vi "Start New File.vi"(8 "error in (no error)":errorcluster, 11 "Logger in":refnum<class "Logger.lvclass">) -> (0 "error out":errorcluster, 2 "File Path":path, 3 "Logger out":refnum<class "Logger.lvclass">)   [LabVIEW 2016, in "Logger.lvclass"]
uses:
  Logger.lvclass
  Logger.lvclass/Logger.ctl
  Read File.lvclass.vi
  Write File.lvclass.vi
  NHMFL_Core/Libraries/File/File Class/File.lvclass
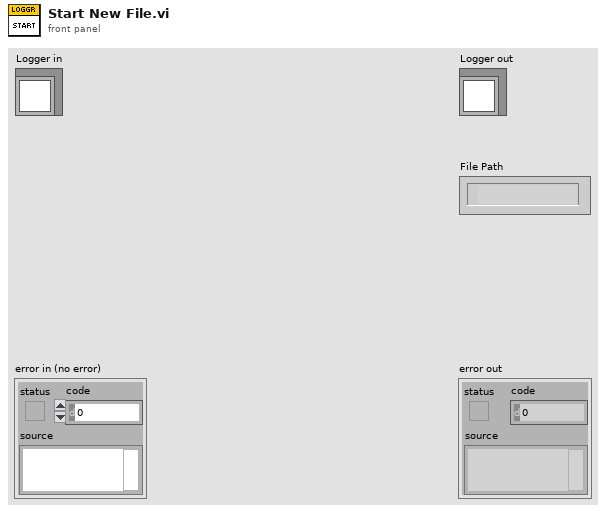
[diagram p1: front panel]
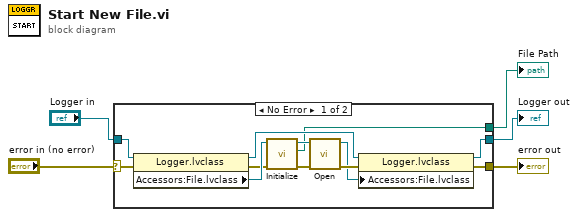
[diagram p0: block diagram]
diagram:
  n1 = case shown="No Error" "error in (no error)" {
    selector: "error in (no error)" -> [w17 w19]
    tunnel: [w12 w19] -> w4
    tunnel: [w11 w18] -> w2
    tunnel: "Logger in" -> [w16 w18]
    tunnel: [w6 _] -> w1
    frame No Error {
      n2 = property class="Logger.lvclass"(reference=w16, error in=w17) -> (reference out=w14:refnum<class "Logger.lvclass">, error out=w13:errorcluster, "Accessors:File.lvclass"=w15:refnum<class "File.lvclass">)
      n3 = call-dynamic "Initialize.vi"("error in (no error)"=w13, "File in"=w15) -> ("error out"=w9:errorcluster, "File Path"=w6:path, "File out"=w10:refnum<class "File.lvclass">)  [unwired: 7 in]
      n4 = call-dynamic "Open.vi"("error in (no error)"=w9, "File in"=w10) -> ("error out"=w8:errorcluster, "File out"=w7:refnum<class "File.lvclass">)  [unwired: 8 in]
      n5 = property class="Logger.lvclass"(reference=w14, error in=w8, "Accessors:File.lvclass"=w7) -> (reference out=w11:refnum<class "Logger.lvclass">, error out=w12:errorcluster)
    }
    frame Error {
    }
  }
  "error out" <- w4
  "Logger out" <- w2
  "File Path" <- w1
